vi "Combination Test.vi"() -> ()   [LabVIEW 2018]
uses:
  5a9499bb-b307-4a4d-bae3-2140953a7cf6.vi
  api/configuration/handlers/file_handler/File Handler.lvclass
  api/configuration/filters/regex_filter/Regex.lvclass
  api/configuration/filters/regex_filter/New (Element).vi
  api/configuration/filters/combination_filter/Combination.lvclass
  api/extension/filter_interface/Match Behavior.ctl
  api/GLog.lvlib
  api/extension/filter_interface/Aggregation Method.ctl
  api/logger_class/Internal Log Levels.ctl
  api/Log Record.ctl
  api/Failure Information.ctl
panel:
  out "failures info":T1[](array[typedef]) {"Log Record"."timestamp" format="%<%x %.3X>T"}
  out "error out":errorcluster
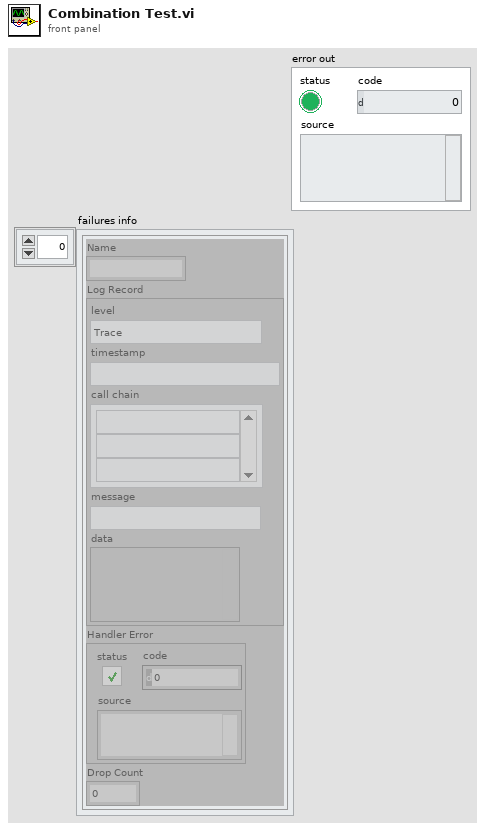
[diagram p1: front panel]
types:
  T1 = typedef "GLog.lvlib/Failure Information.ctl" = cluster{"Name":string, "Log Record":T2, "Handler Error":errorcluster, "Drop Count":u32}
  T2 = typedef "GLog.lvlib/Log Record.ctl" = cluster{"level":T3, "timestamp":timestamp, "call chain":string[], "message":string, "data":variant}
  T3 = typedef "GLog.lvlib/Internal Log Levels.ctl" = enum16{"Trace", "Debug", "Info", "Warning", "Error", "Critical", "Internal"}
  T4 = typedef "GLog.lvlib/Aggregation Method.ctl" = enum16{"Any", "Only", "All", "None"}
  T5 = typedef "GLog.lvlib/Match Behavior.ctl" = enum16{"Keep", "Discard"}
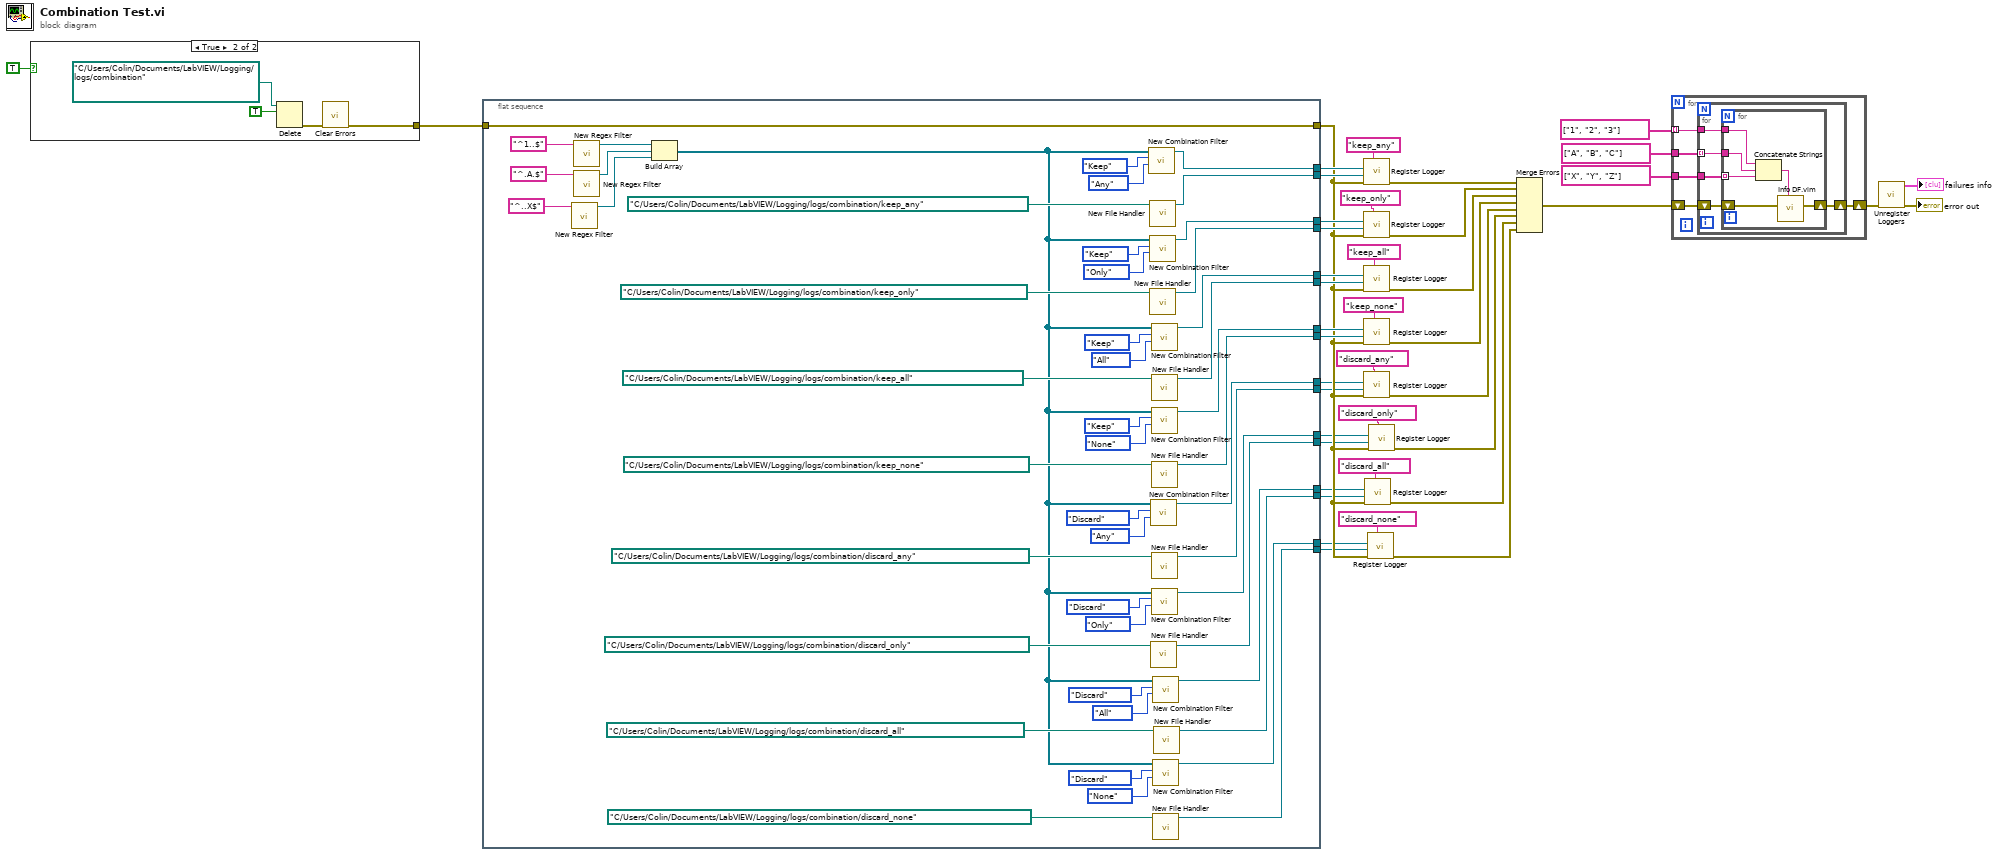
[diagram p0: block diagram]
diagram:
  n1 = case shown="True" TRUE {
    tunnel: [_ w43] -> w37
    frame False {
    }
    frame True {
      n2 = Delete(path (use dialog)=path "C:/Users/Colin/Documents/LabVIEW/Logging/logs/combination" ("log directory (<app dir>/logs)"), entire hierarchy (F)=TRUE) -> (error out=w45:errorcluster)  [unwired: 3 in, 2 out]
      n3 = call <vilib>:"Clear Errors.vi"("error in (no error)"=w45) -> ("error out"=w43:errorcluster)  [unwired: 5 in, 1 out]
    }
  }
  n4 = flat-sequence {
    tunnel: [w93] -> w42
    tunnel: w37 -> [w90]
    tunnel: [w90] -> w12
    tunnel: [w61] -> w33
    tunnel: [w60] -> w26
    tunnel: [w59] -> w25
    tunnel: [w58] -> w24
    tunnel: [w57] -> w23
    tunnel: [w56] -> w22
    tunnel: [w55] -> w21
    tunnel: [w54] -> w11
    tunnel: [w53] -> w10
    tunnel: [w52] -> w9
    tunnel: [w51] -> w8
    tunnel: [w50] -> w7
    tunnel: [w49] -> w6
    tunnel: [w48] -> w5
    tunnel: [w47] -> w4
    frame #0 {
      n5 = call-poly "New Regex Filter.vi"("regex string"="^..X$") -> ("regex out"=w86:refnum<class "Regex.lvclass">)  [unwired: 9 in, 1 out]
      n6 = call-poly "New Regex Filter.vi"("regex string"="^1..$") -> ("regex out"=w88:refnum<class "Regex.lvclass">)  [unwired: 9 in, 1 out]
      n7 = call-poly "New Regex Filter.vi"("regex string"="^.A.$") -> ("regex out"=w87:refnum<class "Regex.lvclass">)  [unwired: 9 in, 1 out]
      n8 = Build Array(w88, w87, w86) -> (w62:refnum<class "Regex.lvclass">[])
      n9 = call "New Combination Filter.vi"("aggregation method (any)"=Aggregation_Method."Any", "match behavior (keep)"=Match_Behavior."Keep", "sub-filters"=w62) -> ("aggregate filter"=w61:refnum<class "Combination.lvclass">)  [unwired: 8 in]
      n10 = call "New File Handler.vi"("log directory (<app dir>/logs)"=path "C:/Users/Colin/Documents/LabVIEW/Logging/logs/combination/keep_any") -> ("file handler"=w93:refnum<class "File Handler.lvclass">)  [unwired: 10 in]
      n11 = call "New Combination Filter.vi"("aggregation method (any)"=Aggregation_Method."Only", "match behavior (keep)"=Match_Behavior."Keep", "sub-filters"=w62) -> ("aggregate filter"=w60:refnum<class "Combination.lvclass">)  [unwired: 8 in]
      n12 = call "New File Handler.vi"("log directory (<app dir>/logs)"=path "C:/Users/Colin/Documents/LabVIEW/Logging/logs/combination/keep_only") -> ("file handler"=w59:refnum<class "File Handler.lvclass">)  [unwired: 10 in]
      n13 = call "New Combination Filter.vi"("aggregation method (any)"=Aggregation_Method."Any", "match behavior (keep)"=Match_Behavior."Discard", "sub-filters"=w62) -> ("aggregate filter"=w54:refnum<class "Combination.lvclass">)  [unwired: 8 in]
      n14 = call "New File Handler.vi"("log directory (<app dir>/logs)"=path "C:/Users/Colin/Documents/LabVIEW/Logging/logs/combination/discard_only") -> ("file handler"=w51:refnum<class "File Handler.lvclass">)  [unwired: 10 in]
      n15 = call "New Combination Filter.vi"("aggregation method (any)"=Aggregation_Method."All", "match behavior (keep)"=Match_Behavior."Keep", "sub-filters"=w62) -> ("aggregate filter"=w58:refnum<class "Combination.lvclass">)  [unwired: 8 in]
      n16 = call "New Combination Filter.vi"("aggregation method (any)"=Aggregation_Method."None", "match behavior (keep)"=Match_Behavior."Keep", "sub-filters"=w62) -> ("aggregate filter"=w56:refnum<class "Combination.lvclass">)  [unwired: 8 in]
      n17 = call "New File Handler.vi"("log directory (<app dir>/logs)"=path "C:/Users/Colin/Documents/LabVIEW/Logging/logs/combination/keep_none") -> ("file handler"=w55:refnum<class "File Handler.lvclass">)  [unwired: 10 in]
      n18 = call "New File Handler.vi"("log directory (<app dir>/logs)"=path "C:/Users/Colin/Documents/LabVIEW/Logging/logs/combination/discard_any") -> ("file handler"=w53:refnum<class "File Handler.lvclass">)  [unwired: 10 in]
      n19 = call "New Combination Filter.vi"("aggregation method (any)"=Aggregation_Method."Only", "match behavior (keep)"=Match_Behavior."Discard", "sub-filters"=w62) -> ("aggregate filter"=w52:refnum<class "Combination.lvclass">)  [unwired: 8 in]
      n20 = call "New File Handler.vi"("log directory (<app dir>/logs)"=path "C:/Users/Colin/Documents/LabVIEW/Logging/logs/combination/keep_all") -> ("file handler"=w57:refnum<class "File Handler.lvclass">)  [unwired: 10 in]
      n21 = call "New Combination Filter.vi"("aggregation method (any)"=Aggregation_Method."All", "match behavior (keep)"=Match_Behavior."Discard", "sub-filters"=w62) -> ("aggregate filter"=w50:refnum<class "Combination.lvclass">)  [unwired: 8 in]
      n22 = call "New Combination Filter.vi"("aggregation method (any)"=Aggregation_Method."None", "match behavior (keep)"=Match_Behavior."Discard", "sub-filters"=w62) -> ("aggregate filter"=w48:refnum<class "Combination.lvclass">)  [unwired: 8 in]
      n23 = call "New File Handler.vi"("log directory (<app dir>/logs)"=path "C:/Users/Colin/Documents/LabVIEW/Logging/logs/combination/discard_none") -> ("file handler"=w47:refnum<class "File Handler.lvclass">)  [unwired: 10 in]
      n24 = call "New File Handler.vi"("log directory (<app dir>/logs)"=path "C:/Users/Colin/Documents/LabVIEW/Logging/logs/combination/discard_all") -> ("file handler"=w49:refnum<class "File Handler.lvclass">)  [unwired: 10 in]
    }
  }
  n25 = call "Register Logger.vi"("name (\"Default\")"="keep_any" ("name (\"Default\")"), "error in (no error)"=w12, "log handler (file handler)"=w42, "log filter (none)"=w33) -> ("error out"=w41:errorcluster)  [unwired: 7 in]
  n26 = call "Register Logger.vi"("name (\"Default\")"="keep_only" ("name (\"Default\")"), "error in (no error)"=w12, "log handler (file handler)"=w25, "log filter (none)"=w26) -> ("error out"=w32:errorcluster)  [unwired: 7 in]
  n27 = call "Register Logger.vi"("name (\"Default\")"="keep_all" ("name (\"Default\")"), "error in (no error)"=w12, "log handler (file handler)"=w23, "log filter (none)"=w24) -> ("error out"=w29:errorcluster)  [unwired: 7 in]
  n28 = call "Register Logger.vi"("name (\"Default\")"="keep_none" ("name (\"Default\")"), "error in (no error)"=w12, "log handler (file handler)"=w21, "log filter (none)"=w22) -> ("error out"=w28:errorcluster)  [unwired: 7 in]
  n29 = call "Register Logger.vi"("name (\"Default\")"="discard_any" ("name (\"Default\")"), "error in (no error)"=w12, "log handler (file handler)"=w10, "log filter (none)"=w11) -> ("error out"=w20:errorcluster)  [unwired: 7 in]
  n30 = call "Register Logger.vi"("name (\"Default\")"="discard_all" ("name (\"Default\")"), "error in (no error)"=w12, "log handler (file handler)"=w6, "log filter (none)"=w7) -> ("error out"=w15:errorcluster)  [unwired: 7 in]
  n31 = call "Register Logger.vi"("name (\"Default\")"="discard_none" ("name (\"Default\")"), "error in (no error)"=w12, "log handler (file handler)"=w4, "log filter (none)"=w5) -> ("error out"=w14:errorcluster)  [unwired: 7 in]
  n32 = call "Register Logger.vi"("name (\"Default\")"="discard_only" ("name (\"Default\")"), "error in (no error)"=w12, "log handler (file handler)"=w8, "log filter (none)"=w9) -> ("error out"=w18:errorcluster)  [unwired: 7 in]
  n33 = Merge Errors(w41, w32, w29, w28, w20, w18, w15, w14) -> (w39:errorcluster)
  n34 = for {
    shift-right: [w98] -> w3
    shift-left: w39 -> [w99]
    tunnel: string[] ["1", "2", "3"] -> [w97] mode=indexing
    tunnel: string[] ["A", "B", "C"] -> [w96]
    tunnel: string[] ["X", "Y", "Z"] -> [w95]
    n35 = for {
      shift-right: [w103] -> w98
      shift-left: w99 -> [w104]
      tunnel: w97 -> [w102]
      tunnel: w96 -> [w101] mode=indexing
      tunnel: w95 -> [w100]
      n36 = for {
        shift-right: [w109] -> w103
        shift-left: w104 -> [w110]
        tunnel: w102 -> [w108]
        tunnel: w101 -> [w107]
        tunnel: w100 -> [w106] mode=indexing
        n37 = Concatenate Strings(w108, w107, w106) -> (w105:string)
        n38 = call "Info DF.vim"("message"=w105, "dataflow in"=w110) -> ("dataflow out"=w109:errorcluster)  [unwired: 9 in]
      }
    }
  }
  n39 = call "Unregister Loggers.vi"("error in (no error)"=w3) -> ("error out"=→"error out":errorcluster, "failures info"=→"failures info":T1[])  [unwired: 9 in]
